vi "Device PPL Folder.vi"(8 "error in (no error)":errorcluster, 11 "Device in":refnum<class "Device.lvclass">) -> (0 "error out":errorcluster, 1 "class path":path, 2 "vi path":path, 3 "Relative Class Path":path)   [LabVIEW 2020, in "HAL.lvlib" / "Device.lvclass"]
uses:
  Device.lvclass
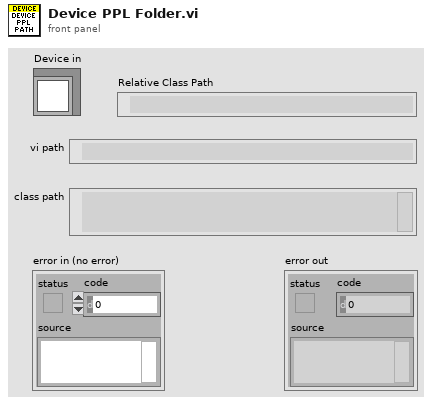
[diagram p1: front panel]
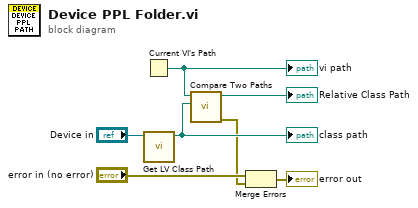
[diagram p0: block diagram]
diagram:
  n1 = Current VI's Path() -> (path=w3:path)
  "vi path" <- w3
  n2 = call <vilib>:"Get LV Class Path.vi"("object"="Device in") -> ("class path"=w4:path)  [unwired: 9 in, 1 out]
  "class path" <- w4
  n3 = call <vilib>:"Compare Two Paths.vi"("Path 2"=w4, "Path 1"=w3) -> ("error out"=w1:errorcluster, "Relative Path from 1 to 2"=→"Relative Class Path":path)  [unwired: 6 in, 2 out]
  n4 = Merge Errors("error in (no error)", w1) -> (→"error out":errorcluster)
